vi "Read FW Version (No Objects).vi"(8 "errorIN":errorcluster, 11 "LCD in":T1) -> (0 "error out":errorcluster, 1 "FW Version":dbl, 3 "LCD out":T1)   [LabVIEW 2012]
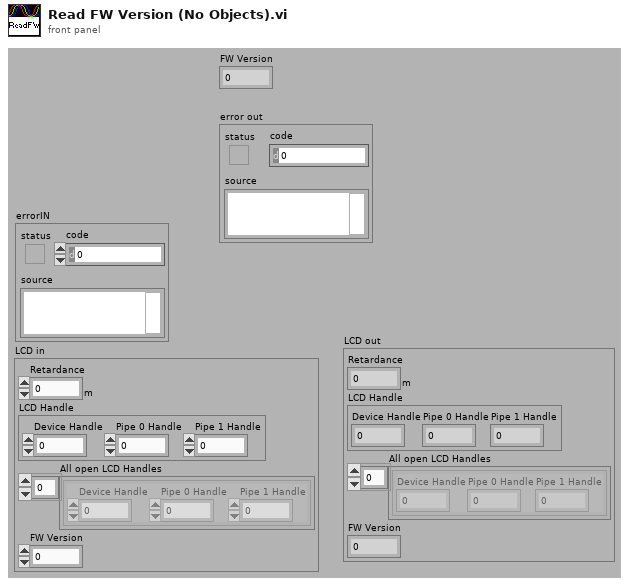
[diagram p1: front panel]
types:
  T1 = cluster{"Retardance":dbl[unit], "LCD Handle":cluster{"Device Handle":u32, "Pipe 0 Handle":u32, "Pipe 1 Handle":u32}, "All open LCD Handles":cluster{"Device Handle":u32, "Pipe 0 Handle":u32, "Pipe 1 Handle":u32}[], "FW Version":dbl}
  T2 = cluster{"Device Handle":u32, "Pipe 0 Handle":u32, "Pipe 1 Handle":u32}
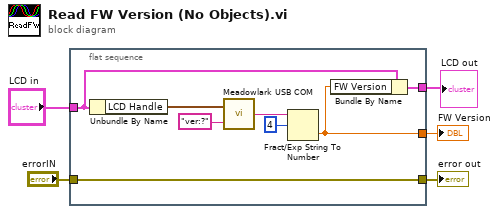
[diagram p0: block diagram]
diagram:
  n1 = flat-sequence {
    tunnel: [w6] -> w3
    tunnel: [w7] -> w2
    tunnel: "LCD in" -> [w9]
    tunnel: "errorIN" -> [w10]
    tunnel: [w10] -> w5
    frame #0 {
      n2 = Unbundle By Name(w9) -> ("LCD Handle"=w8:T2)
      n3 = call "Meadowlark USB COM.vi"("WRITE IN String"="ver:?", "USB Open Device Cluster"=w8) -> ("READ OUT String"=w11:string)
      n4 = Fract/Exp String To Number(string=w11, offset=4) -> (number=w6:dbl)  [unwired: 3 out]
      n5 = Bundle By Name(cluster=w9, "FW Version"=w6) -> (w7:T1)
    }
  }
  "error out" <- w5
  "FW Version" <- w3
  "LCD out" <- w2
